vi "NumBy1E6.vi"(11 "Double":dbl) -> (3 "Numeric":dbl)   [LabVIEW 2018]
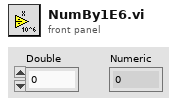
[diagram p1: front panel]
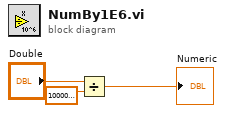
[diagram p0: block diagram]
diagram:
  n1 = Divide(x="Double", y=1000000.0) -> (x/y=→"Numeric":dbl)
